vi "Register panel as running.vi"(8 "error in (no error)":errorcluster, 10 "\"This VI\" reference from current panel":refnum<vi>, 11 "Fiber Auto Collimation panel in":refnum<class "Fiber Auto Collimation panel.lvclass">) -> (0 "error out":errorcluster, 3 "Fiber Auto Collimation panel out":refnum<class "Fiber Auto Collimation panel.lvclass">)   [LabVIEW 2018, in "Fiber Auto Collimation panel.lvclass"]
doc: "Registers a Panel as \"running\". Should only be called on the Panel VI itself, never externally. It should be called once at the start of the panel after event registration is completed but before the main loop(s), and then never again (unless the panel stops and restarts, of course).\n\nAfter the \"running\" registration is complete, the panel is set to be shown unless the \"Start hidden\" Boolean was earlier set to be True.\n\nThe input for \"This VI\" as a reference means a reference to the panel VI itself, in case it needs to be manipulated (for instance, placed into a sub-panel).\n\nThe \"clone name\" property should have been set in the static wrapper that called the panel, and any other settings in the private data of the class should be set before calling this VI as well.\n\nThis VI attempts to run regardless of any input errors."
uses:
  Fiber Auto Collimation panel.lvclass
  Fiber Auto Collimation panel.lvclass/Fiber Auto Collimation panel.ctl
  6b8e813c-30ca-4a5d-b77a-9de90d2a83bd.vi
  <userlib>/nLight Error Handling/Merge errors no loss.vi
  References/Fiber Auto Collimation References.lvclass
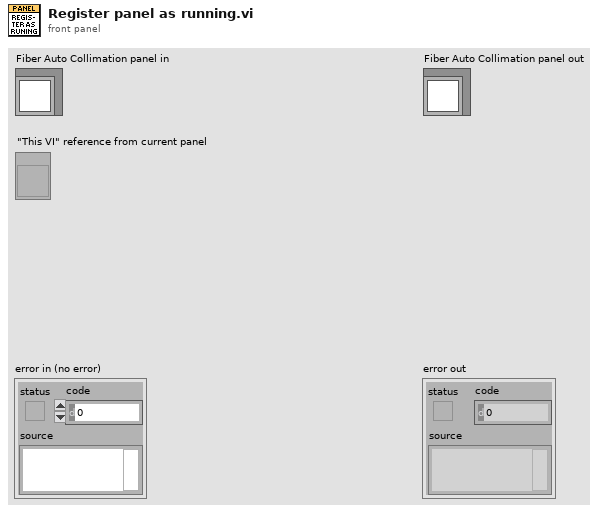
[diagram p1: front panel]
types:
  T1 = enum32{"Invalid", "Standard", "Closed", "Hidden", "Minimized", "Maximized"}
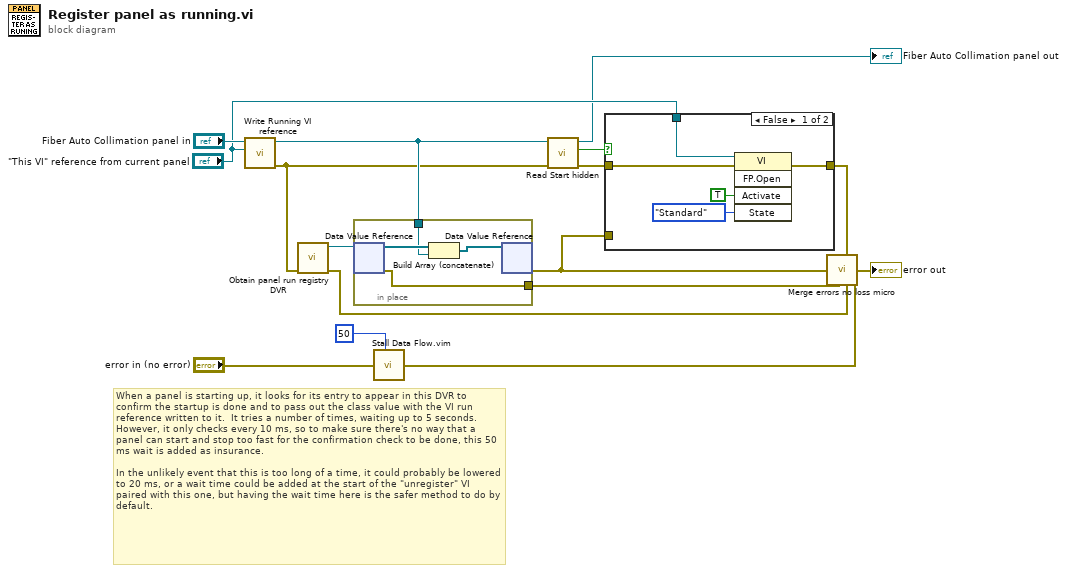
[diagram p0: block diagram]
diagram:
  # "When a panel is starting up, it looks for its entry to appear in this DVR to confirm the startup is done and to pass out the class value with the VI run reference written to it.  It tries a number of times, waiting up to 5 seconds.  However, it only checks every 10 ms, so to make sure there's no way that a panel can start and stop too fast for the confirmation check to be done, this 50 ms wait is added as insurance.\n\nIn the unlikely event that this is too long of a time, it could probably be lowered to 20 ms, or a wait time could be added at the start of the \"unregister\" VI paired with this one, but having the wait time here is the safer method to do by default."
  n1 = call "Write Running VI reference.vi"("Running VI reference"="\"This VI\" reference from current panel", "Fiber Auto Collimation panel in"="Fiber Auto Collimation panel in") -> ("error out"=w1:errorcluster, "Fiber Auto Collimation panel out"=w6:refnum<class "Fiber Auto Collimation panel.lvclass">)  [unwired: 8 in]
  n2 = call "Obtain panel run registry DVR.vi"("error in"=w1) -> ("error out"=w12:errorcluster, "Panel registration DVR"=w16:refnum<data-value>)  [unwired: 9 in]
  n3 = in-place {
    in-place-border: w6 -> [w19]
    in-place-border: [w17] -> w13
    n4 = in-place-dvr #1(w16) -> (w20:refnum<class "Fiber Auto Collimation panel.lvclass">[], w17:errorcluster)
    n5 = Build Array (concatenate)(w20, w19) -> (w18:refnum<class "Fiber Auto Collimation panel.lvclass">[])
    n6 = in-place-dvr #1(w18) -> (w2:errorcluster)  [unwired: 1 out]
  }
  n7 = call "Stall Data Flow.vim"("value in"="error in (no error)", "milliseconds to wait"=u32 50) -> ("value out"=w10:errorcluster)  [unwired: 1 out]
  n8 = call "Read Start hidden.vi"("error in (no error)"=w1, "Fiber Auto Collimation panel in"=w6) -> ("error out"=w7:errorcluster, "Start hidden"=w3:bool, "Fiber Auto Collimation panel out"=→"Fiber Auto Collimation panel out":refnum<class "Fiber Auto Collimation panel.lvclass">)  [unwired: 7 in]
  n9 = case shown="False" w3 {
    tunnel: "\"This VI\" reference from current panel" -> [w25 _]
    tunnel: w7 -> [w24 w26]
    tunnel: [w23 w26] -> w4
    tunnel: w2 -> [_ _]
    frame False {
      n10 = invoke class="VI" method="FP.Open"(reference=w25, error in=w24, "Activate"=TRUE ("Activate?"), "State"=T1."Standard") -> (error out=w23:errorcluster)  [unwired: 1 in, 4 out]
    }
    frame True {
    }
  }
  n11 = call <userlib>:"Merge errors no loss micro.vi"("error in (no error) 1"=w2, "error in (no error) 5"=w13, "error in (no error) 3"=w4, "error in (no error) 6"=w12, "error in (no error) 7"=w10) -> ("error out"=→"error out":errorcluster)  [unwired: 4 in]
